vi "VI Tree.vi"   [LabVIEW 2018, in "Zurich Instruments LabOne.lvlib"]
doc: "This is the instrument driver for the <INSTRUMENT NAME>. The VI Tree displays all the user-callable VIs of the instrument driver in an organized table."
uses:
  Zurich Instruments LabOne.lvlib
  Configure/ziGetValueDouble.vi
  Configure/ziSetValueDouble.vi
  Modules/ziModSetValueBinary.vi
  Modules/ziModGetDoubleData.vi
  Utility/ziTicksToS_single.vi
  Data/ziGetEventAuxInSample.vi
  Modules/ziModGetNodeValueDouble.vi
panel:
  # "(c) 2009-2014 Zurich Instruments.  ALL RIGHTS RESERVED."
  # "SEE DIAGRAM\nFOR VI TREE."
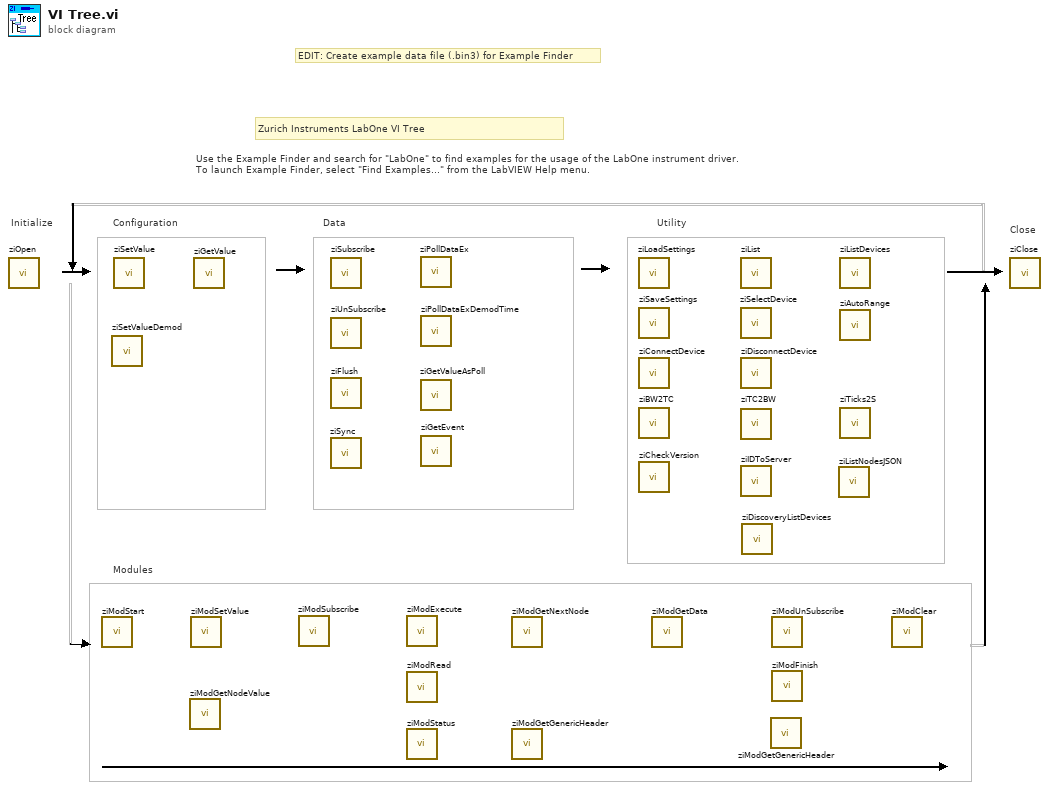
[diagram p0: block diagram]
diagram:
  # "Modules"
  # "Zurich Instruments LabOne VI Tree"
  # "EDIT: Create example data file (.bin3) for Example Finder"
  # "Use the Example Finder and search for \"LabOne\" to find examples for the usage of the LabOne instrument driver.\nTo launch Example Finder, select \"Find Examples...\" from the LabVIEW Help menu."
  # "Configuration"
  # "Utility"
  # "Data"
  # "Close"
  # "Initialize"
  n1 = call "ziOpen.vi"() -> ()  [unwired: 4 in, 3 out]
  n2 = call "ziModStart.vi"() -> ()  [unwired: 9 in, 3 out]
  n3 = call "ziSetValueDemod.vi"() -> ()  [unwired: 10 in, 2 out]
  n4 = call-poly "ziSetValue.vi"() -> ()  [unwired: 5 in, 2 out]
  n5 = call-poly "ziModGetNodeValue.vi"() -> ()  [unwired: 13 in, 3 out]
  n6 = call-poly "ziModSetValue.vi"() -> ()  [unwired: 10 in, 2 out]
  n7 = call-poly "ziGetValue.vi"() -> ()  [unwired: 3 in, 3 out]
  n8 = call "ziModSubscribe.vi"() -> ()  [unwired: 9 in, 2 out]
  n9 = call "ziSubscribe.vi"() -> ()  [unwired: 4 in, 2 out]
  n10 = call "ziUnSubscribe.vi"() -> ()  [unwired: 4 in, 2 out]
  n11 = call "ziFlush.vi"() -> ()  [unwired: 10 in, 2 out]
  n12 = call "ziSync.vi"() -> ()  [unwired: 14 in, 2 out]
  n13 = call "ziModExecute.vi"() -> ()  [unwired: 8 in, 3 out]
  n14 = call "ziModRead.vi"() -> ()  [unwired: 10 in, 2 out]
  n15 = call "ziModStatus.vi"() -> ()  [unwired: 7 in, 4 out]
  n16 = call "ziPollDataEx.vi"() -> ()  [unwired: 4 in, 8 out]
  n17 = call "ziPollDataExDemodTime.vi"() -> ()  [unwired: 9 in, 3 out]
  n18 = call "ziGetValueAsPoll.vi"() -> ()  [unwired: 4 in, 2 out]
  n19 = call-poly "ziGetEvent.vi"() -> ()  [unwired: 9 in, 3 out]
  n20 = call "ziModGetNextNode.vi"() -> ()  [unwired: 8 in, 4 out]
  n21 = call "ziModGetGenericHeader.vi"() -> ()  [unwired: 9 in, 3 out]
  n22 = call "ziLoadSettings.vi"() -> ()  [unwired: 5 in, 2 out]
  n23 = call "ziSaveSettings.vi"() -> ()  [unwired: 4 in, 3 out]
  n24 = call "ziConnectDevice.vi"() -> ()  [unwired: 10 in, 2 out]
  n25 = call "ziBW2TC.vi"() -> ()  [unwired: 3 in, 1 out]
  n26 = call "ziCheckVersion.vi"() -> ()  [unwired: 13 in, 3 out]
  n27 = call-poly "ziModGetData.vi"() -> ()  [unwired: 7 in, 5 out]
  n28 = call "ziList.vi"() -> ()  [unwired: 4 in, 3 out]
  n29 = call "ziSelectDevice.vi"() -> ()  [unwired: 3 in, 3 out]
  n30 = call "ziDisconnectDevice.vi"() -> ()  [unwired: 10 in, 2 out]
  n31 = call "ziTC2BW.vi"() -> ()  [unwired: 3 in, 1 out]
  n32 = call "ziIDToServer.vi"() -> ()  [unwired: 13 in, 3 out]
  n33 = call "ziDiscoveryListDevices.vi"() -> ()  [unwired: 9 in, 3 out]
  n34 = call "ziModGetGenericHeader.vi"() -> ()  [unwired: 9 in, 3 out]
  n35 = call "ziModUnSubscribe.vi"() -> ()  [unwired: 10 in, 2 out]
  n36 = call "ziModFinish.vi"() -> ()  [unwired: 9 in, 2 out]
  n37 = call "ziListNodesJSON.vi"() -> ()  [unwired: 13 in, 3 out]
  n38 = call "ziListDevices.vi"() -> ()  [unwired: 5 in, 3 out]
  n39 = call "ziAutoRange.vi"() -> ()  [unwired: 9 in, 3 out]
  n40 = call-poly "ziTicks2S.vi"() -> ()  [unwired: 3 in, 3 out]
  n41 = call "ziModClear.vi"() -> ()  [unwired: 9 in, 2 out]
  n42 = call "ziClose.vi"() -> ()  [unwired: 4 in, 2 out]
